vi "Dig Grave Practice.vi"(11 "Input":bool[](array[boolean])=[FALSE, FALSE, FALSE, TRUE, FALSE, FALSE]) -> (3 "Any?":bool)   [LabVIEW 2017, in "Tests.lvlib"]
uses:
  Tests.lvlib
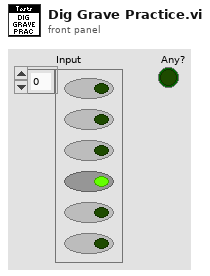
[diagram p1: front panel]
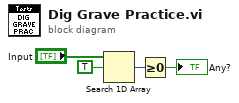
[diagram p0: block diagram]
diagram:
  n1 = Search 1D Array(1D array="Input", element=TRUE) -> (index of element=w2:i32)  [unwired: 1 in]
  n2 = Greater Or Equal To 0?(x=w2) -> (x >= 0?=→"Any?":bool)
